vi "Error Read.vi"(8 "error in":errorcluster, 11 "Climate Chamber in":refnum<class "Climate Chamber.lvclass">) -> (0 "error out":errorcluster, 1 "Changed or First Call?":bool, 2 "Error ACT":bool, 3 "Climate Chamber out":refnum<class "Climate Chamber.lvclass">)   [LabVIEW 2023, in "Climate Chamber.lvclass"]
uses:
  Climate Chamber.lvclass
  Climate Chamber.lvclass/Climate Chamber.ctl
  Low Level Capabilities/Error/Error.lvclass
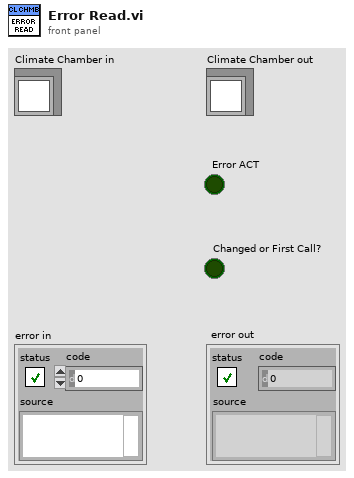
[diagram p1: front panel]
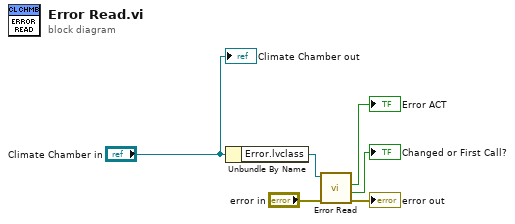
[diagram p0: block diagram]
diagram:
  n1 = Unbundle By Name("Climate Chamber in") -> ("Error.lvclass"=w6:refnum<class "Error.lvclass">)
  n2 = call-dynamic "Error Read.vi"("error in"="error in", "Error in"=w6) -> ("error out"=→"error out":errorcluster, "Changed or First Call?"=→"Changed or First Call?":bool, "Error ACT"=→"Error ACT":bool)  [unwired: 6 in, 1 out]
  "Climate Chamber out" <- "Climate Chamber in"
